vi "AI_Select_CheckBox.vi"(10 "Checkbox Cluster":T2={"Boolean"=TRUE, "Boolean 2"=TRUE, "Boolean 3"=TRUE, "Boolean 4"=TRUE, "Boolean 5"=FALSE, "Boolean 6"=FALSE, "Boolean 7"=FALSE, "Boolean 8"=FALSE}) -> ()   [LabVIEW 2013]
panel:
  in  "AI Configuration":T1(array[cluster])=[{"AI.Coupling"=10050, "AI.Max"=0.1, "AI.Min"=-0.1, "Input physical channels"="PXI2Slot6/ai0:1"}] {"AI.Coupling" items=["AC"=10045, "DC"=10050, "GND"=10066]}
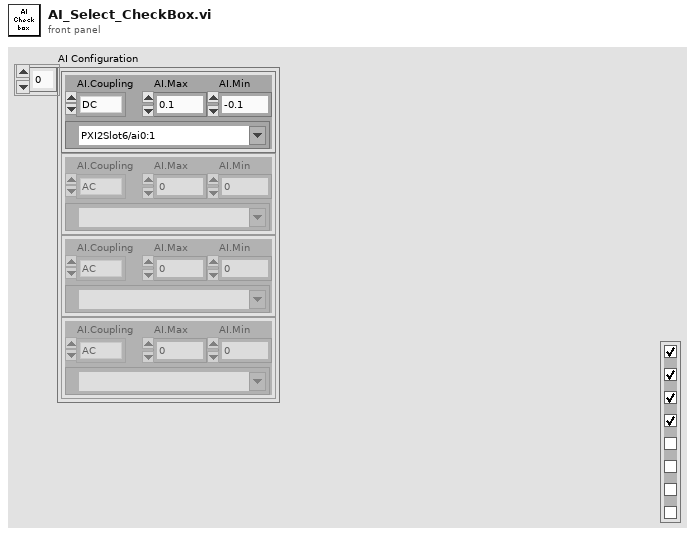
[diagram p1: front panel]
types:
  T1 = cluster{"AI.Coupling":i32, "AI.Max":dbl, "AI.Min":dbl, "Input physical channels":tag}[]
  T2 = cluster{"Boolean":bool, "Boolean 2":bool, "Boolean 3":bool, "Boolean 4":bool, "Boolean 5":bool, "Boolean 6":bool, "Boolean 7":bool, "Boolean 8":bool}
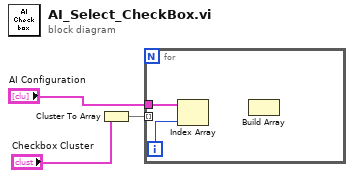
[diagram p0: block diagram]
diagram:
  n1 = Cluster To Array(cluster="Checkbox Cluster") -> (array=w3:bool[])
  n2 = for {
    tunnel: "AI Configuration" -> [w4]
    tunnel: w3 -> [_] mode=indexing
    i -> [w5]
    n3 = Index Array(array=w4, index=w5) -> ()  [unwired: 1 out]
    n4 = Build Array() -> ()  [unwired: 2 in, 1 out]
  }
